vi "ValChange.vi"(6 "Value":string, 7 "Col Array Ref in":refnum<vi>, 8 "error in (no error)":errorcluster, 9 "Table CtlRef In":refnum<vi>, 10 "Cell Position":T1, 11 "MenuCol in":refnum<class "MenuCol.lvclass">) -> (0 "error out":errorcluster, 1 "Table CtlRef Out":refnum<vi>, 3 "MenuCol out":refnum<class "MenuCol.lvclass">)   [LabVIEW 2013, in "MenuCol.lvclass"]
doc: "If a table cell value changes, calling this method will ensure the change is pushed down to any subsequent disabled cells.\nThis is read only w.r.t. column data (only for dynamic dispatch)."
uses:
  MenuCol.lvclass
  <vilib>/Utility/miscctls.llb/LVRowAndColumnTypeDef.ctl
  Column/Column.lvclass/Column.ctl
  Column/Column.lvclass
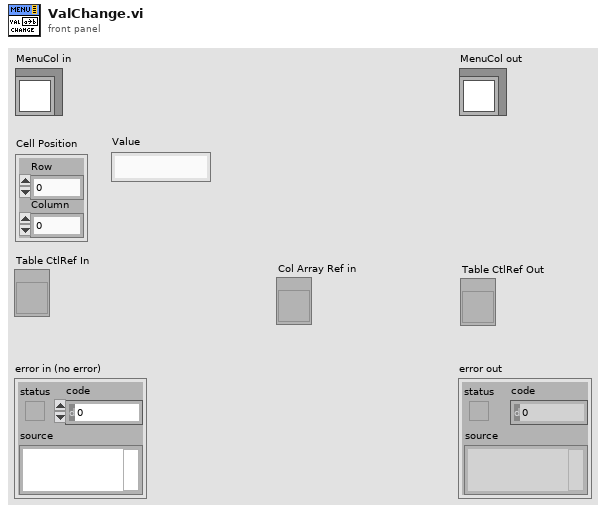
[diagram p1: front panel]
types:
  T1 = typedef "LVRowAndColumnTypeDef.ctl" = cluster{"Row":i32, "Column":i32}
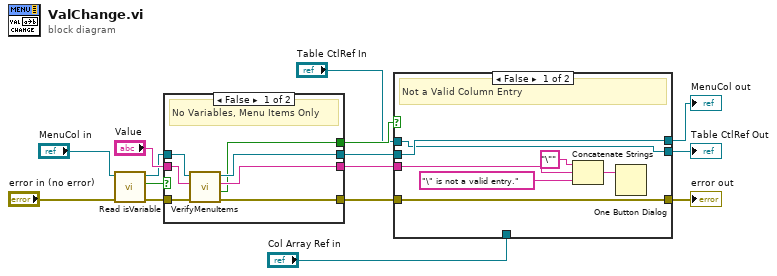
[diagram p0: block diagram]
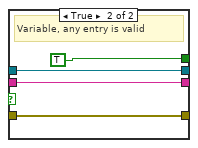
[diagram p2: hidden frame]
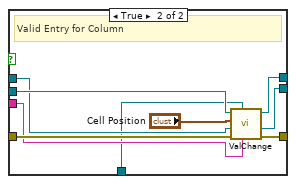
[diagram p3: hidden frame]
diagram:
  n1 = call "Read isVariable.vi"("error in (no error)"="error in (no error)", "Column in"="MenuCol in") -> ("error out"=w11:errorcluster, "isVariable?"=w10:bool, "Column out"=w14:refnum<class "MenuCol.lvclass">)  [unwired: 7 in]
  n2 = case shown="False" w10 {
    tunnel: "Value" -> [w22 w23]
    tunnel: [w21 w23] -> w8
    tunnel: [w20 w25] -> w7
    tunnel: [w19 w24] -> w6
    tunnel: [w18 TRUE ("Unknown Menu Item")] -> w9
    tunnel: w14 -> [w17 w25]
    tunnel: w11 -> [w16 w24]
    frame False {
      # "No Variables, Menu Items Only"
      n3 = call-dynamic "VerifyMenuItems.vi"("error in (no error)"=w16, "Menu Item In"=w22, "MenuCol in"=w17) -> ("error out"=w19:errorcluster, "Valid Menu Item"=w18:bool, "Menu Item Out"=w21:string, "MenuCol out"=w20:refnum<class "MenuCol.lvclass">)  [unwired: 5 in]
    }
    frame True {
      # "Variable, any entry is valid"
    }
  }
  n4 = case shown="False" w9 {
    tunnel: w8 -> [w27 w35]
    tunnel: w7 -> [w33 w42]
    tunnel: w6 -> [w31 w41]
    tunnel: [w31 w40] -> w4
    tunnel: [w32 w39] -> w3
    tunnel: [w33 w38] -> w2
    tunnel: "Table CtlRef In" -> [w32 w37]
    tunnel: "Col Array Ref in" -> [_ w34]
    frame False {
      # "Not a Valid Column Entry"
      n5 = Concatenate Strings("\"" ("string"), w27, "\" is not a valid entry." ("string")) -> (w30:string)
      n6 = One Button Dialog(message=w30) -> ()  [unwired: 1 in, 1 out]
    }
    frame True {
      # "Valid Entry for Column"
      n7 = call-parent "ValChange.vi"("Value"=w35, "Col Array Ref in"=w34, "error in (no error)"=w41, "Table CtlRef In"=w37, "Cell Position"="Cell Position", "Column in"=w42) -> ("error out"=w40:errorcluster, "Table CtlRef Out"=w39:refnum<vi>, "Column out"=w38:refnum<class "MenuCol.lvclass">)  [unwired: 3 in]
    }
  }
  "error out" <- w4
  "MenuCol out" <- w2
  "Table CtlRef Out" <- w3
